vi "ChirpSourceGen(SubVI).vi"(3 "Frequency2(Hz)":dbl=30000.0 format="%#_6p", 4 "Frequency1(Hz)":dbl=30000.0 format="%#_6p", 5 "Pulse length(sec)":dbl=30000.0 format="%#_6p", 6 "Fs(Hz)":dbl=30000.0 format="%#_6p") -> (0 "dt":dbl, 1 "M.F. Tap(F2-1)":dbl[](array[numeric]), 2 "M.F. Tap(F1-2)":dbl[](array[numeric]))   [LabVIEW 2017]
uses:
  <vilib>/Analysis/NI_AALBase.lvlib
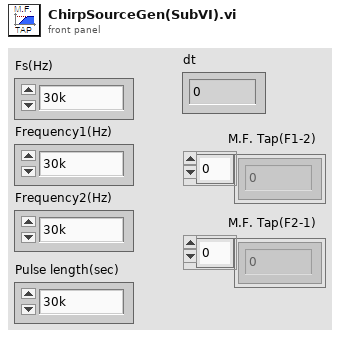
[diagram p1: front panel]
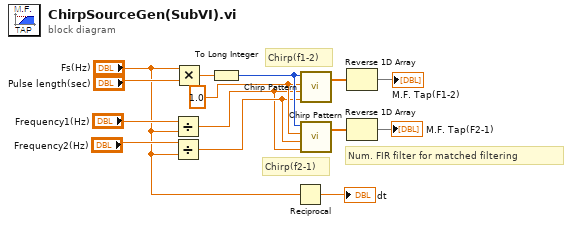
[diagram p0: block diagram]
diagram:
  w8 = 1.0 ("amplitude")
  # "Num. FIR filter for matched filtering"
  # "Chirp(f2-1)"
  # "Chirp(f1-2)"
  n1 = Divide(x="Frequency1(Hz)", y="Fs(Hz)") -> (x/y=w6:dbl)
  n2 = Divide(x="Frequency2(Hz)", y="Fs(Hz)") -> (x/y=w7:dbl)
  n3 = Multiply(x="Fs(Hz)", y="Pulse length(sec)") -> (x*y=w13:dbl)
  n4 = To Long Integer(number=w13) -> (32bit integer=w9:i32)
  n5 = Reciprocal(x="Fs(Hz)") -> (1/x=→"dt":dbl)
  n6 = call <vilib>:"Chirp Pattern.vi"("f2"=w7, "f1"=w6, "amplitude"=w8, "samples"=w9) -> ("Chirp Pattern"=w12:dbl[])  [unwired: 1 out]
  n7 = call <vilib>:"Chirp Pattern.vi"("f2"=w6, "f1"=w7, "amplitude"=w8, "samples"=w9) -> ("Chirp Pattern"=w5:dbl[])  [unwired: 1 out]
  n8 = Reverse 1D Array(array=w12) -> (reversed array=→"M.F. Tap(F1-2)":dbl[])
  n9 = Reverse 1D Array(array=w5) -> (reversed array=→"M.F. Tap(F2-1)":dbl[])
